vi "Mono (YJ).vi"(3 "error in (no error)":errorcluster, 5 "Go to Wavelength":dbl, 6 "CmdLib In":refnum<k24>) -> (0 "error out 2":errorcluster, 1 "State of Mono_SetWavelength":bool=TRUE, 2 "Current Wavelength":dbl)   [LabVIEW 2017]
uses:
  C:/Users/Admin/Desktop/Sensitive EQE Stuff/S-EQE (YJ)/Mono vi (YJ)/Cornerstone.dll
  Cornerstone.dll
panel:
  out "Numeric":i32
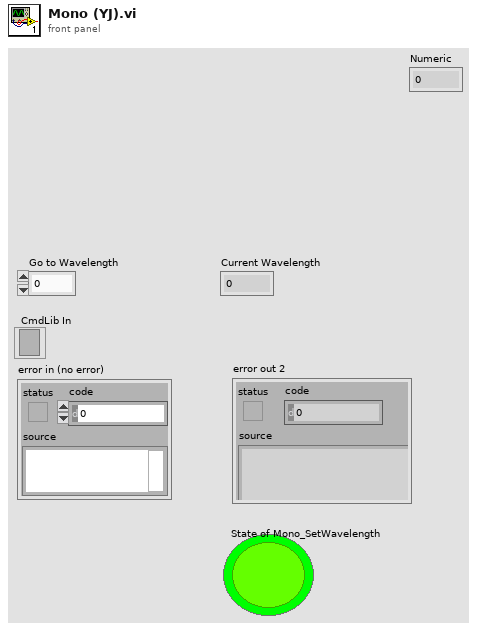
[diagram p1: front panel]
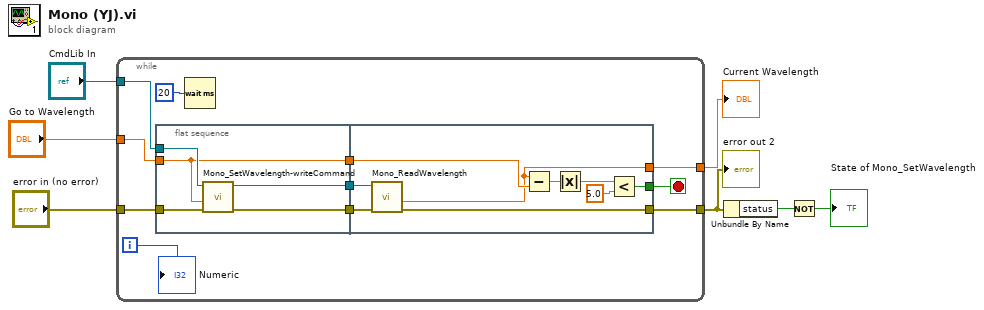
[diagram p0: block diagram]
diagram:
  n1 = while {
    tunnel: "error in (no error)" -> [w13]
    tunnel: "CmdLib In" -> [w12]
    tunnel: [w11] -> w5
    tunnel: [w10] -> w2
    tunnel: "Go to Wavelength" -> [w9]
    i -> [w8]
    stop <- w15 stop-if-true
    n2 = flat-sequence {
      tunnel: [w22] -> w18
      tunnel: [w21] -> w17
      tunnel: [w19] -> w16
      tunnel: w13 -> [w23]
      tunnel: w12 -> [w20]
      tunnel: w9 -> [w19]
      tunnel: w18 -> [w31]
      tunnel: w17 -> [w32]
      tunnel: w16 -> [w30]
      tunnel: [w26] -> w15
      tunnel: [w25] -> w11
      tunnel: [w24] -> w10
      frame #0 {
        n3 = call "Mono_SetWavelength-writeCommand.vi"("error in (no error) 2"=w23, "Wavelength"=w19, "CmdLib In"=w20) -> ("error out 2"=w22:errorcluster, "CmdLib Out"=w21:refnum<k24>)  [unwired: 6 in, 1 out]
      }
      frame #1 {
        n4 = call "Mono_ReadWavelength.vi"("error in (no error) 2"=w31, "CmdLib In"=w32) -> ("error out 2"=w25:errorcluster, "getWavelength"=w24:dbl)  [unwired: 7 in, 1 out]
        n5 = Subtract(x=w24, y=w30) -> (x-y=w29:dbl)
        n6 = Absolute Value(x=w29) -> (abs(x)=w28:dbl)
        n7 = Less?(x=w28, y=5.0) -> (x < y?=w26:bool)
      }
    }
    n8 = Wait (ms)(milliseconds to wait=u32 20) -> ()  [unwired: 1 out]
    "Numeric" <- w8
  }
  "error out 2" <- w5
  "Current Wavelength" <- w2
  n9 = Unbundle By Name(w5) -> ("status"=w4:bool)
  n10 = Not(x=w4) -> (.not. x?=→"State of Mono_SetWavelength":bool)
